vi "Configure LXI For ARM-Trigger.vi"(0 "VISA resource name":refnum<visa-resource-name>, 1 "Enable LXI Event (T: Enable)":bool=TRUE, 2 "LXI Destination Host Name":string[](array[string]), 3 "LAN Identifier":string[](array[string]), 5 "LXI Event (0: LAN0)":i32(ring) items=["LAN0", "LAN1", "LAN2", "LAN3", "LAN4", "LAN5", "LAN6", "LAN7"], 7 "LXI Event Type (0: ARM)":i32(ring) items=["ARM", "Trigger"], 9 "LXI Event Source (0: WaitingForAcquireArm1)":i32(ring) items=["WaitingForAcquireArm1", "WaitingForTransitionArm1", "WaitingForAcquireArm2", "WaitingForTransitionArm2", "WaitingForAcquireTrigger1", "WaitingForTransitionTrigger1", "WaitingForAcquireTrigger2", "WaitingForTransitionTrigger2", "Measuring1", "Measuring2", "Settling1", "Settling2"], 11 "error in (no error)":errorcluster, 12 "LXI Event Detection (0: Rise)":i32(ring) items=["Rise", "Fall", "High", "Low"], 13 "LXI Destination Port Number":i32[](array[numeric])) -> (4 "VISA resource name out":refnum<visa-resource-name>, 15 "error out":errorcluster)   [LabVIEW 2020, in "Agilent B2900 Series.lvlib"]
doc: "Configures the LXI Trigger Event for trigger layer or ARM layer. \nTo use LXI Triggers, set the trigger source to LAN first. \nCall Configure Trigger Layer.vi or Configure ARM Layer.vi to set the trigger source."
uses:
  Agilent B2900 Series.lvlib
panel:
  # "LXI Event Destination"
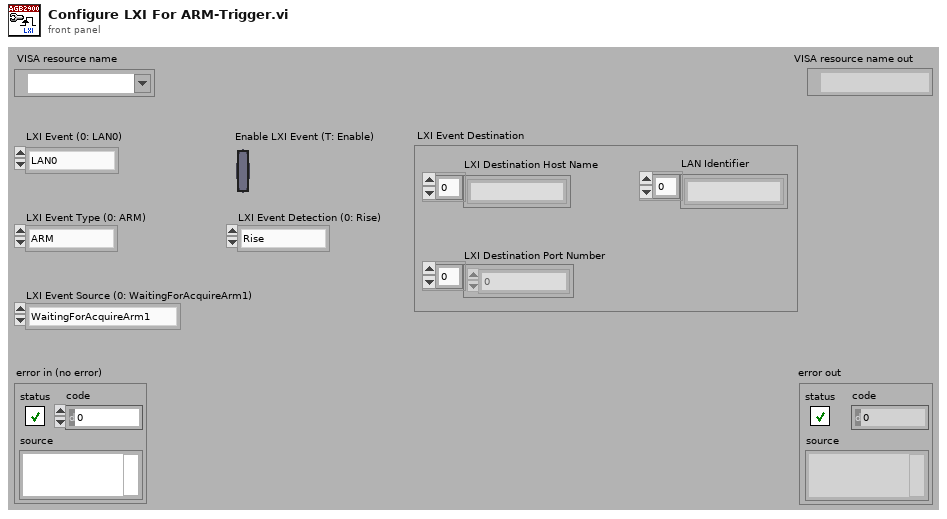
[diagram p1: front panel]
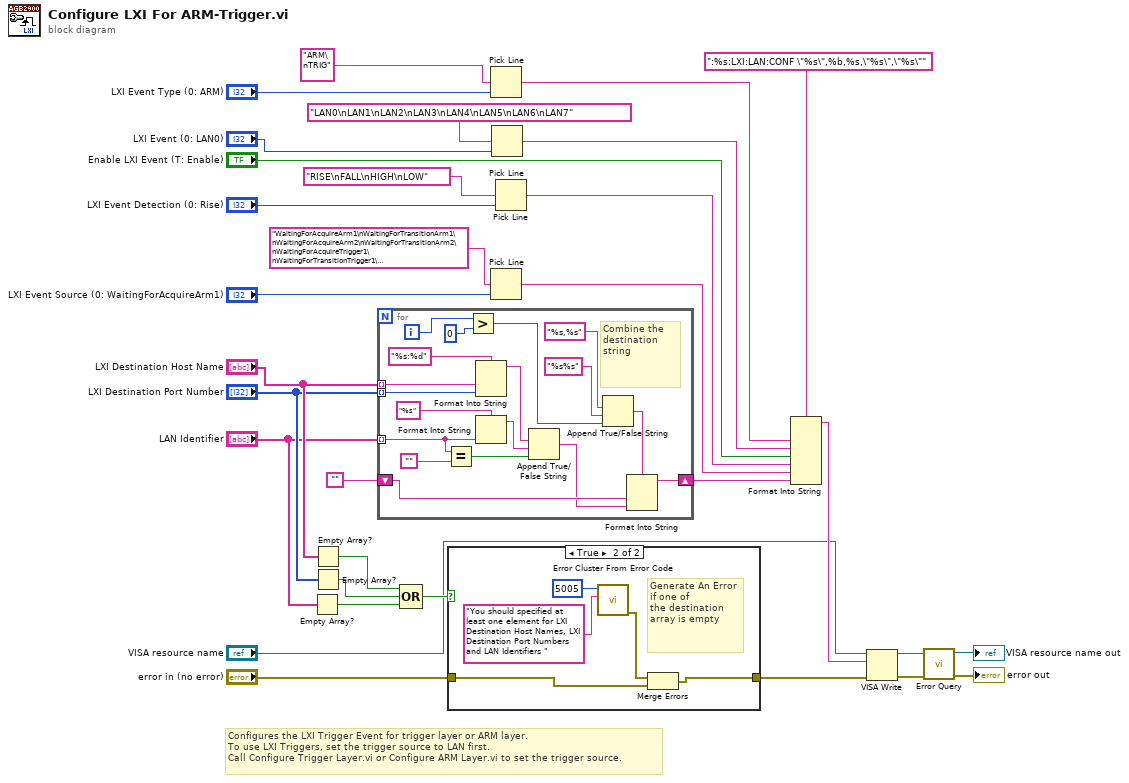
[diagram p0: block diagram]
diagram:
  # "Configures the LXI Trigger Event for trigger layer or ARM layer.  \nTo use LXI Triggers, set the trigger source to LAN first. \nCall Configure Trigger Layer.vi or Configure ARM Layer.vi to set the trigger source."
  n1 = Empty Array?(array="LAN Identifier") -> (empty?=w5:bool)
  n2 = Empty Array?(array="LXI Destination Host Name") -> (empty?=w10:bool)
  n3 = Empty Array?(array="LXI Destination Port Number") -> (empty?=w6:bool)
  n4 = for {
    tunnel: "LXI Destination Host Name" -> [w48] mode=indexing
    tunnel: "LXI Destination Port Number" -> [w47] mode=indexing
    tunnel: "LAN Identifier" -> [w44] mode=indexing
    shift-right: [w32] -> w13
    shift-left: "" ("Empty String Constant") -> [w37]
    i -> [w40]
    # "Combine the destination string"
    n5 = Equal?(x=w44, y="" ("Empty String Constant")) -> (x = y?=w42:bool)
    n6 = Greater?(x=w40, y=0) -> (0:w38:bool)
    n7 = Format Into String(format string="%s:%d", w48, w47) -> (resulting string=w43:string)  [unwired: 2 in, 1 out]
    n8 = Format Into String(format string="%s", w44) -> (resulting string=w41:string)  [unwired: 2 in, 1 out]
    n9 = Append True/False String(1:w42, 2:w41, 3:w43) -> (0:w36:string)  [unwired: 1 in]
    n10 = Append True/False String(1:w38, 2:"%s%s" ("false string"), 3:"%s,%s" ("true string")) -> (0:w33:string)  [unwired: 1 in]
    n11 = Format Into String(format string=w33, w37, w36) -> (resulting string=w32:string)  [unwired: 2 in, 1 out]
  }
  n12 = Compound Arithmetic op=OR(w10, w6, w5) -> (w2:bool)
  n13 = case shown="True" w2 {
    tunnel: [w50 w55] -> w4
    tunnel: "error in (no error)" -> [w50 w53]
    frame False {
    }
    frame True {
      # "Generate An Error if one of\nthe destination array is empty"
      n14 = call <vilib>:"Error Cluster From Error Code.vi"("error message (\"\")"="You should specified at least one element for LXI Destination Host Names, LXI Destination Port Numbers and LAN Identifiers " ("error message (\"\")"), "error code (0)"=5005) -> ("error out"=w54:errorcluster)  [unwired: 7 in]
      n15 = Merge Errors(w54, w53) -> (w55:errorcluster)
    }
  }
  n16 = Pick Line(multi-line string="ARM\nTRIG", line index="LXI Event Type (0: ARM)") -> (output string=w20:string)  [unwired: 1 in]
  n17 = Pick Line(multi-line string="WaitingForAcquireArm1\nWaitingForTransitionArm1\nWaitingForAcquireArm2\nWaitingForTransitionArm2\nWaitingForAcquireTrigger1\nWaitingForTransitionTrigger1\nWaitingForAcquireTrigger2\nWaitingForTransitionTrigger2\nMeasuring1\nMeasuring2\nSettling1\nSettling2", line index="LXI Event Source (0: WaitingForAcquireArm1)") -> (output string=w15:string)  [unwired: 1 in]
  n18 = Pick Line(multi-line string="LAN0\nLAN1\nLAN2\nLAN3\nLAN4\nLAN5\nLAN6\nLAN7", line index="LXI Event (0: LAN0)") -> (output string=w19:string)  [unwired: 1 in]
  n19 = Pick Line(multi-line string="RISE\nFALL\nHIGH\nLOW", line index="LXI Event Detection (0: Rise)") -> (output string=w17:string)  [unwired: 1 in]
  n20 = Format Into String(format string=":%s:LXI:LAN:CONF \"%s\",%b,%s,\"%s\",\"%s\"", w20, w19, "Enable LXI Event (T: Enable)", w17, w15, w13) -> (resulting string=w12:string)  [unwired: 2 in, 1 out]
  n21 = VISA Write(VISA resource name="VISA resource name", write buffer=w12, error in (no error)=w4) -> (VISA resource name out=w24:refnum<visa-resource-name>, error out=w23:errorcluster)  [unwired: 1 out]
  n22 = call "Error Query.vi"("error in (no error)"=w23, "VISA resource name"=w24) -> ("error out"=→"error out":errorcluster, "VISA resource name out"=→"VISA resource name out":refnum<visa-resource-name>)  [unwired: 6 in, 2 out]
